vi "P bar graph.vi"(9 "Final state? (T)":bool=TRUE, 11 "Wire in":T1) -> ()   [LabVIEW 2016]
uses:
  TypeDefs/Circuit Cluster.ctl
  Classes/GateAbst/GateAbst.lvclass
panel:
  out "Probability Bar Graph":cluster{i32[], dbl[]}(graph)
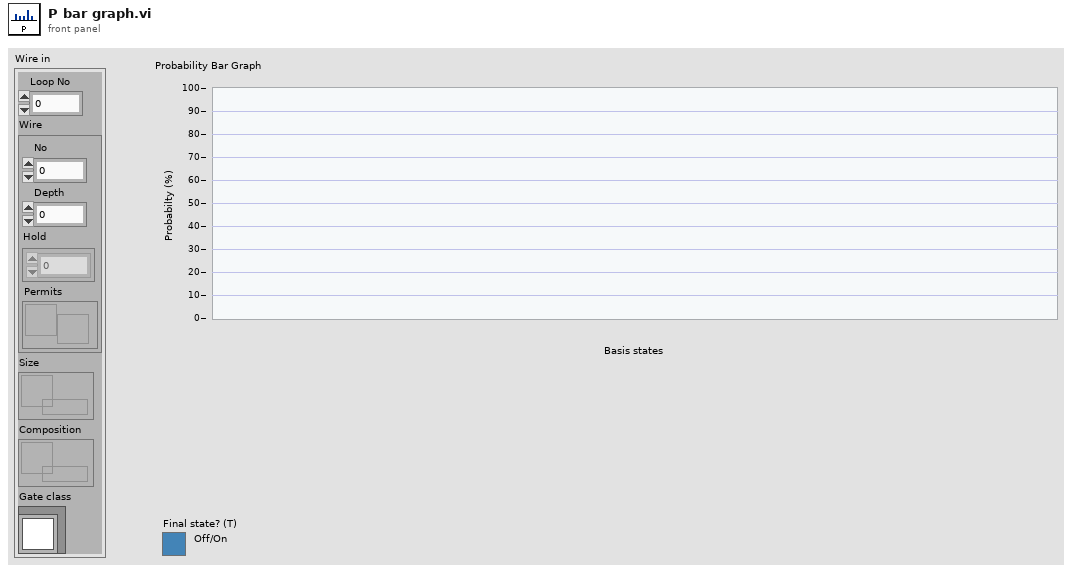
[diagram p1: front panel]
types:
  T1 = typedef "Circuit Cluster.ctl" = cluster{"Loop No":i32, "Wire":cluster{"No":i32, "Depth":i32, "Hold":i32[][], "Permits":refnum<notifier>}, "Size":refnum<queue>, "Composition":refnum<queue>, "Gate class":refnum<class "GateAbst.lvclass">}
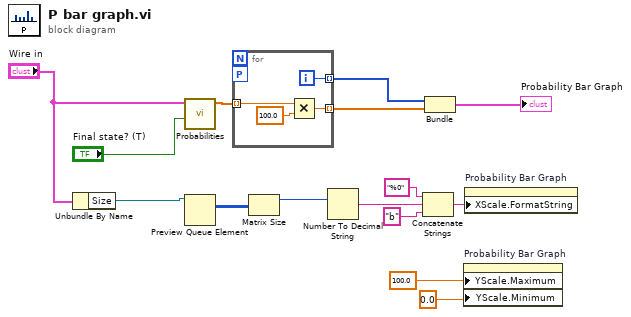
[diagram p0: block diagram]
diagram:
  n1 = Unbundle By Name("Wire in") -> ("Size"=w8:refnum<queue>)
  n2 = call "Probabilities.vi"("Final state? (T)"="Final state? (T)", "Circuit cluster"="Wire in") -> ("Probabilities"=w4:dbl[])  [unwired: 9 in]
  n3 = Preview Queue Element(queue=w8) -> (element=w3:i32[][])  [unwired: 2 in, 3 out]
  n4 = for {
    tunnel: w4 -> [w19] mode=indexing
    tunnel: [w18] -> w15 mode=indexing
    tunnel: [w16] -> w14 mode=indexing
    workers-P: _ -> [_]
    i -> [w16]
    n5 = Multiply(x=w19, y=100.0) -> (x*y=w18:dbl)
  }
  n6 = Matrix Size(0:w3) -> (1:w2:i32)  [unwired: 1 out]
  n7 = Number To Decimal String(number=w2) -> (decimal integer string=w10:string)  [unwired: 1 in]
  n8 = Concatenate Strings("%0" ("string"), w10, "b" ("string")) -> (w9:string)
  n9 = Bundle(w14, w15) -> (→"Probability Bar Graph":cluster{i32[], dbl[]})  [unwired: 1 in]
  n10 = property on="Probability Bar Graph" class="XYGraph (strict)"("YScale.Maximum"=100.0 ("Y Scale.Range:Maximum"), "YScale.Minimum"=0.0 ("Y Scale.Range:Minimum")) -> ()  [unwired: 2 in, 2 out]
  n11 = property on="Probability Bar Graph" class="XYGraph (strict)"("XScale.FormatString"=w9) -> ()  [unwired: 2 in, 2 out]
